vi "dfd_Get NPR Cosine-Modulated Prototype Filter Coefficients.vi"(6 "gama":dbl, 7 "number of bands":i32, 8 "error in (no error)":errorcluster, 10 "roll off":dbl, 11 "initial h":dbl[](array[numeric])) -> (0 "error out":errorcluster, 3 "h":dbl[](array[numeric]))   [LabVIEW 2017, in "NI_DigFilter_FilterBank.lvlib"]
uses:
  <vilib>/addons/Digital Filter Design/NI_DigFilter_FilterBank.lvlib
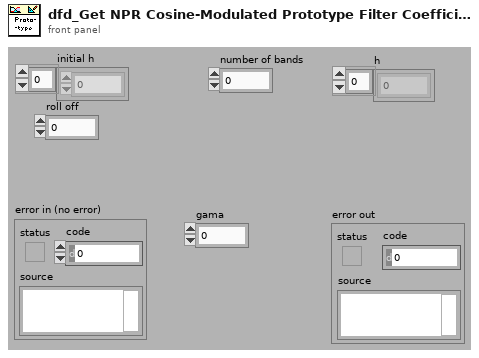
[diagram p1: front panel]
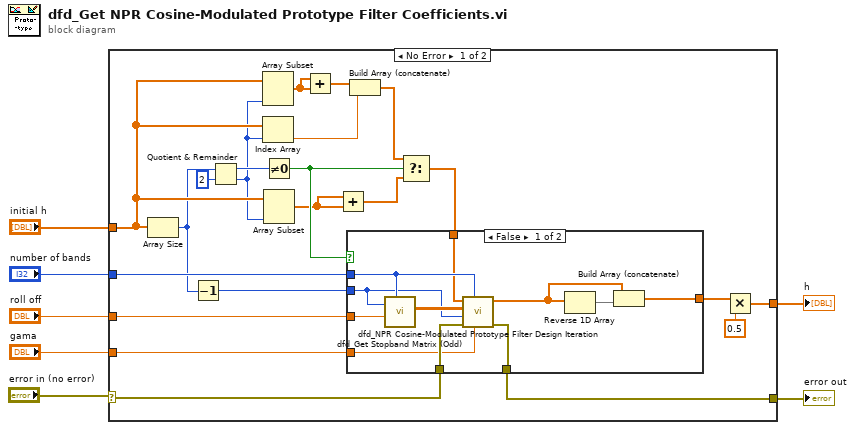
[diagram p0: block diagram]
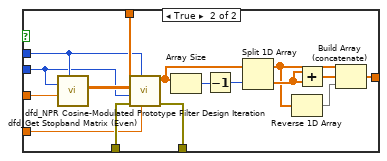
[diagram p2: hidden frame]
diagram:
  n1 = case shown="No Error" "error in (no error)" {
    selector: "error in (no error)" -> [w26 w57]
    tunnel: "gama" -> [w24 _]
    tunnel: [w9 _] -> w6
    tunnel: "roll off" -> [w28 _]
    tunnel: "number of bands" -> [w27 _]
    tunnel: "initial h" -> [w20 _]
    tunnel: [w25 w57] -> w1
    frame No Error {
      n2 = Array Size(array=w20) -> (size(s)=w17:i32)
      n3 = Decrement(x=w17) -> (x-1=w16:i32)
      n4 = Quotient & Remainder(x=w17, y=2) -> (x-y*floor(x/y)=w21:i32, floor(x/y)=w15:i32)
      n5 = Array Subset(array=w20, length=w15) -> (w10:dbl[])  [unwired: 1 in]
      n6 = Index Array(array=w20, index=w15) -> (element=w14:dbl)
      n7 = Not Equal To 0?(x=w21) -> (x != 0?=w18:bool)
      n8 = Array Subset(array=w20, length=w15) -> (w12:dbl[])  [unwired: 1 in]
      n9 = Add(x=w10, y=w10) -> (x+y=w11:dbl[])
      n10 = Add(x=w12, y=w12) -> (x+y=w13:dbl[])
      n11 = Build Array (concatenate)(w11, w14) -> (w23:dbl[])
      n12 = Select(t=w23, s=w18, f=w13) -> (s? t:f=w19:dbl[])
      n13 = case shown="False" w18 {
        tunnel: [w30 w41] -> w29
        tunnel: w28 -> [w39 w54]
        tunnel: w27 -> [w38 w52]
        tunnel: w19 -> [w37 w53]
        tunnel: w26 -> [w35 w46]
        tunnel: [w34 w45] -> w25
        tunnel: w24 -> [w33 w44]
        tunnel: w16 -> [w31 w42]
        frame False {
          n14 = call <vilib>:"dfd_Get Stopband Matrix (Odd).vi"("number of bands"=w38, "roll off"=w39, "order"=w31) -> ("Us"=w32:dbl[][])  [unwired: 8 in]
          n15 = call <vilib>:"dfd_NPR Cosine-Modulated Prototype Filter Design Iteration.vi"("gama"=w33, "number of bands"=w38, "error in (no error)"=w35, "order"=w31, "Us"=w32, "half initial h"=w37) -> ("error out"=w34:errorcluster, "half h"=w36:dbl[])  [unwired: 4 in]
          n16 = Reverse 1D Array(array=w36) -> (reversed array=w40:dbl[])
          n17 = Build Array (concatenate)(w36, w40) -> (w30:dbl[])
        }
        frame True {
          n18 = call <vilib>:"dfd_Get Stopband Matrix (Even).vi"("number of bands"=w52, "roll off"=w54, "order"=w42) -> ("Us"=w43:dbl[][])  [unwired: 8 in]
          n19 = call <vilib>:"dfd_NPR Cosine-Modulated Prototype Filter Design Iteration.vi"("gama"=w44, "number of bands"=w52, "error in (no error)"=w46, "order"=w42, "Us"=w43, "half initial h"=w53) -> ("error out"=w45:errorcluster, "half h"=w51:dbl[])  [unwired: 4 in]
          n20 = Array Size(array=w51) -> (size(s)=w56:i32)
          n21 = Decrement(x=w56) -> (x-1=w55:i32)
          n22 = Split 1D Array(array=w51, index=w55) -> (first subarray=w49:dbl[], second subarray=w50:dbl[])
          n23 = Reverse 1D Array(array=w49) -> (reversed array=w48:dbl[])
          n24 = Add(x=w50, y=w50) -> (x+y=w47:dbl[])
          n25 = Build Array (concatenate)(w49, w47, w48) -> (w41:dbl[])
        }
      }
      n26 = Multiply(x=w29, y=0.5) -> (x*y=w9:dbl[])
    }
    frame Error {
    }
  }
  "h" <- w6
  "error out" <- w1
